vi "Make HTTP Request v4.vi"(0 "HTTP-Verb":string(combo)="GET", 3 "URL Prefix":string, 4 "URL Suffix":string, 5 "error in":errorcluster, 6 "request headers":T1[](array[typedef])=[{"name"="Content-Type", "value"="application/x-amz-json-1.1"}], 7 "request parameters":T1[](array[typedef]), 9 "request body":string, 10 "AWS Core":refnum<class "NI_AWS_Core.lvclass">) -> (12 "Call Result":string, 14 "response headers":string, 16 "response body":string, 19 "error out":errorcluster)   [LabVIEW 2015, in "NI_AWS_Core.lvclass"]
uses:
  NI_AWS_Core.lvclass
  Name Value Pair.ctl
  NI_AWS_Core.lvclass/NI_AWS_Core.ctl
  Read Credentials.vi
  Read Service.vi
  Read Region.vi
  Read Verify Server.vi
  <vilib>/httpClient/LabVIEWHTTPClient.lvlib
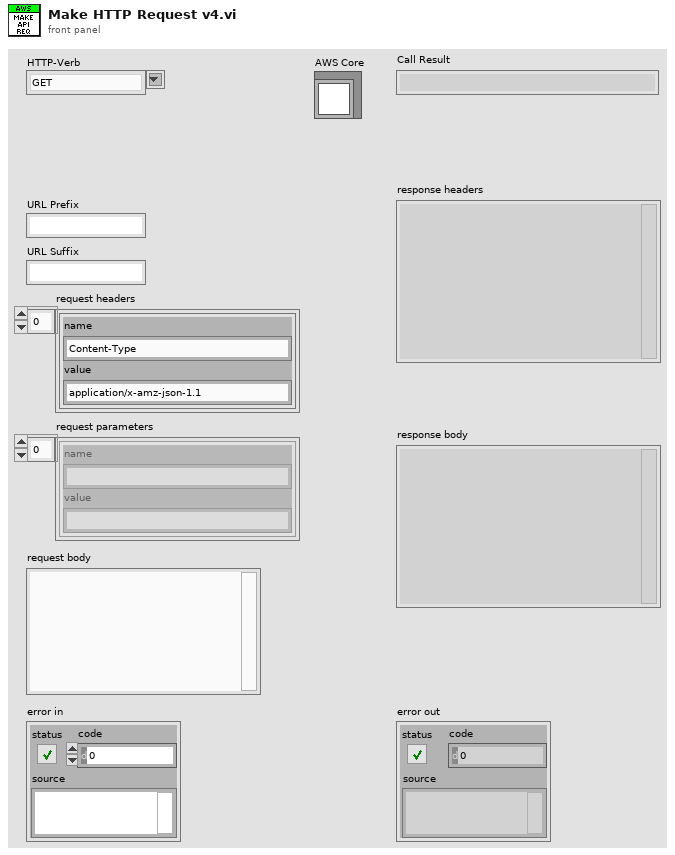
[diagram p1: front panel]
types:
  T1 = typedef "NI_AWS_Core.lvclass/Name Value Pair.ctl" = cluster{"name":string, "value":string}
  T2 = typedef "AWS Core.lvlib/AWS Credentials.ctl" = cluster{"Access Key":string, "Secret Key":string}
  T3 = typedef "NI_AWS Core.lvlib/Region.ctl" = enum16{"us-east-1", "us-east-2", "us-west-1", "us-west-2", "ap-northeast-1", "ap-northeast-2", "ap-southeast-1", "ap-southeast-2", "ca-central-1", "eu-central-1", "eu-west-1", "eu-west-2", "sa-east-1"}
  T4 = typedef "LabVIEWHTTPClient.lvlib/ClientHandle.ctl" = refnum<k1>
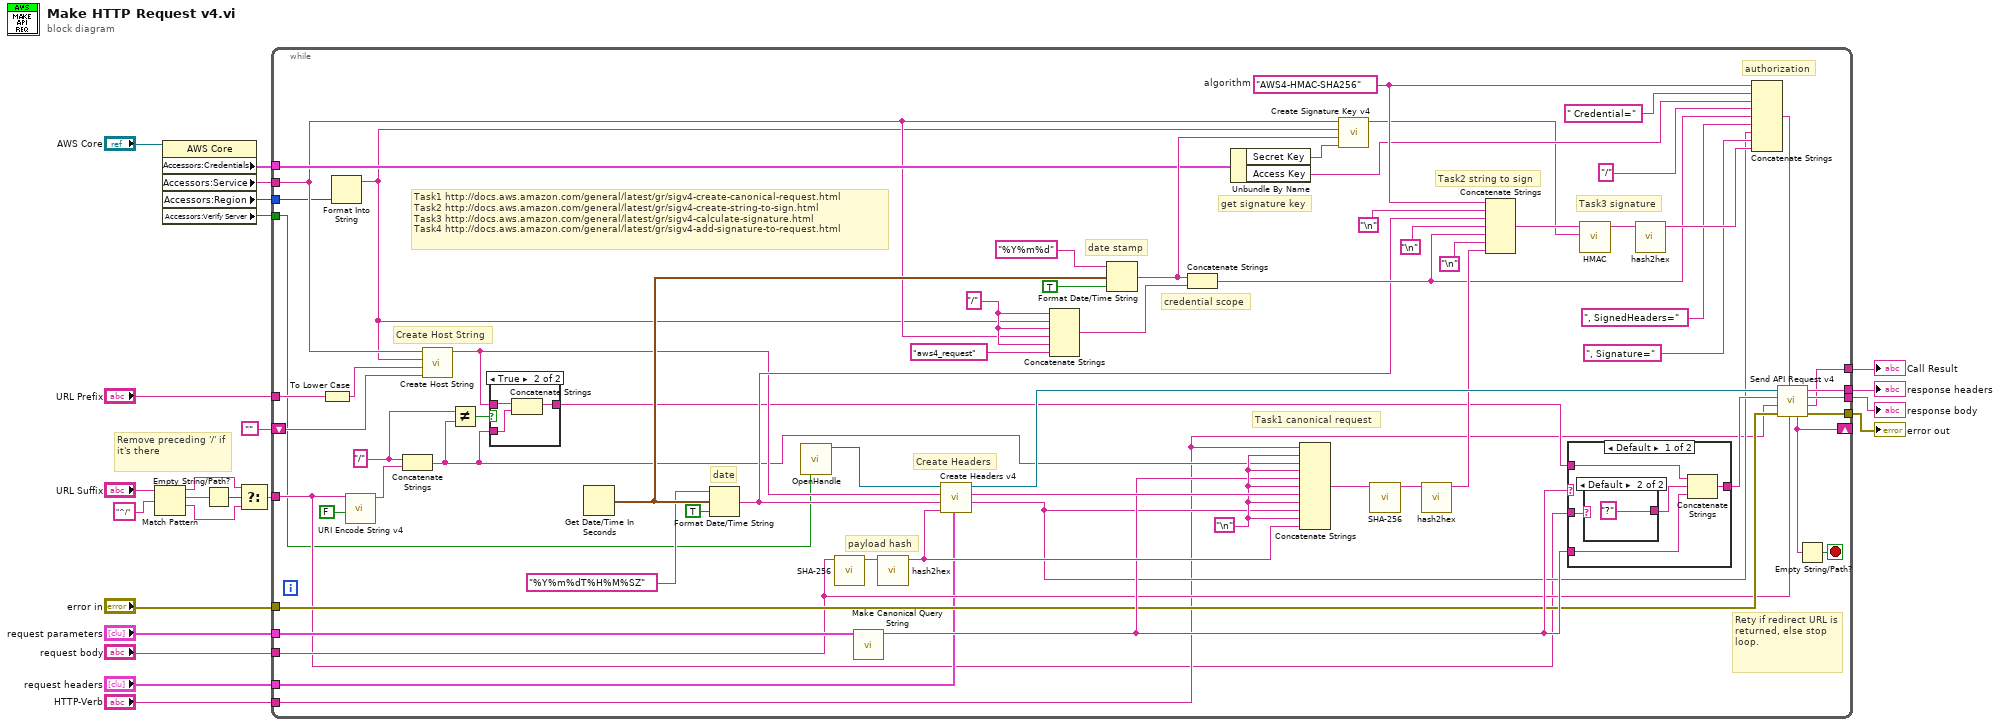
[diagram p0: block diagram]
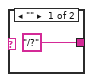
[diagram p3: hidden frame]
diagram:
  # "Remove preceding '/' if it's there"
  n1 = Match Pattern(string="URL Suffix", regular expression="^/") -> (before substring=w17:string, match substring=w15:string, after substring=w18:string)  [unwired: 1 in, 1 out]
  n2 = property class="AWS Core"(reference="AWS Core") -> ("Accessors:Credentials"=w5:T2, "Accessors:Service"=w3:string, "Accessors:Region"=w2:T3, "Accessors:Verify Server"=w1:bool)  [unwired: 1 in, 2 out]
  n3 = Empty String/Path?(string/path=w15) -> (empty?=w16:bool)
  n4 = Select(t=w17, s=w16, f=w18) -> (s? t:f=w13:string)
  n5 = while {
    tunnel: [w88] -> w23
    tunnel: [w41] -> w21
    tunnel: [w46] -> w20
    shift-right: [w45] -> _
    shift-left: "" ("Redirect endpoint") -> [w43]
    tunnel: [w42] -> w22
    tunnel: "error in" -> [w38]
    tunnel: w13 -> [w28]
    tunnel: "URL Prefix" -> [w34]
    tunnel: "request parameters" -> [w33]
    tunnel: "request body" -> [w32]
    tunnel: "request headers" -> [w31]
    tunnel: "HTTP-Verb" -> [w30]
    tunnel: w5 -> [w29]
    tunnel: w3 -> [w27]
    tunnel: w2 -> [w25]
    tunnel: w1 -> [w26]
    stop <- w44 stop-if-true
    w51 = "/" ("string")
    w62 = "/" ("string")
    w80 = "AWS4-HMAC-SHA256"  # algorithm
    w58 = "\n"
    # "Rety if redirect URL is returned, else stop loop."
    # "Create Host String"
    # "Task1 canonical request"
    # "Create Headers"
    # "get signature key"
    # "Task1 http://docs.aws.amazon.com/general/latest/gr/sigv4-create-canonical-request.html\nTask2 http://docs.aws.amazon.com/general/latest/gr/sigv4-create-string-to-sign.html\nTask3 http://docs.aws.amazon.com/general/latest/gr/sigv4-calculate-signature.html\nTask4 http://docs.aws.amazon.com/general/latest/gr/sigv4-add-signature-to-request.html"
    # "date stamp"
    # "date"
    # "payload hash"
    # "authorization"
    # "Task3 signature"
    # "Task2 string to sign"
    # "credential scope"
    n6 = To Lower Case(string=w34) -> (all lower case string=w39:string)
    n7 = Format Into String(w25) -> (resulting string=w24:string)  [unwired: 3 in, 1 out]
    n8 = call "URI Encode String v4.vi"("Encode /"=FALSE, "Un-encoded String"=w28) -> ("UriEncoded String"=w36:string)  [unwired: 9 in]
    n9 = Concatenate Strings(w51, w36) -> (w48:string)
    n10 = call "Create Host String.vi"("Redirect Endpoint"=w43, "URL Prefix"=w39, "Region"=w24, "AWS Service"=w27) -> ("Host String"=w49:string)  [unwired: 7 in]
    n11 = Not Equal?(x=w51, y=w48) -> (x != y?=w50:bool)
    n12 = case shown="True" w50 {
      tunnel: w49 -> [w89 w92]
      tunnel: w48 -> [_ w91]
      tunnel: [w89 w90] -> w47
      frame False {
      }
      frame True {
        n13 = Concatenate Strings(w92, w91) -> (w90:string)
      }
    }
    n14 = Get Date/Time In Seconds() -> (seconds since 1Jan1904=w55:timestamp)
    n15 = Format Date/Time String(time format string (%c)="%Y%m%dT%H%M%SZ", seconds (now)=w55, UTC format=TRUE) -> (date/time string=w56:string)
    n16 = call <vilib>:"OpenHandle.vi"("verify server(true)"=w26) -> ("client handle out"=w59:T4)  [unwired: 13 in, 1 out]
    n17 = call "SHA-256.vi"("Message"=w32) -> ("Hash Value"=w72:string)  [unwired: 10 in]
    n18 = call "Make Canonical Query String.vi"("request parameters"=w33) -> ("canonical parameters"=w52:string)  [unwired: 10 in]
    n19 = call "hash2hex.vi"("hash string"=w72) -> ("hex string"=w57:string)  [unwired: 10 in]
    n20 = call "Create Headers v4.vi"("request headers"=w31, "RequestBody Payload"=w57, "date/time string"=w56, "Host"=w49, "Client Handle In"=w59) -> ("Signed Headers"=w40:string, "canonical headers"=w76:string, "Client Handle Out"=w86:T4)  [unwired: 3 in]
    n21 = Concatenate Strings(w62, w24, w62, w27, w62, "aws4_request" ("string")) -> (w63:string)
    n22 = Format Date/Time String(time format string (%c)="%Y%m%d", seconds (now)=w55, UTC format=TRUE) -> (date/time string=w69:string)
    n23 = Concatenate Strings(w69, w63) -> (w64:string)
    n24 = Unbundle By Name(w29) -> ("Secret Key"=w60:string, "Access Key"=w66:string)
    n25 = Concatenate Strings(w30, w58, w48, w58, w52, w58, w76, w58, w40, w58, w57) -> (w71:string)
    n26 = call "Create Signature Key v4.vi"("AWS Service"=w27, "Region"=w24, "date/time string"=w69, "Secret Key"=w60) -> ("Keyed-Hash"=w37:string)  [unwired: 6 in]
    n27 = call "SHA-256.vi"("Message"=w71) -> ("Hash Value"=w70:string)  [unwired: 10 in]
    n28 = call "hash2hex.vi"("hash string"=w70) -> ("hex string"=w79:string)  [unwired: 10 in]
    n29 = Concatenate Strings(w80, "\n", w56, "\n", w64, "\n", w79) -> (w68:string)
    n30 = case shown="Default" w52 {
      tunnel: [w97 w100] -> w53
      tunnel: w47 -> [w95 w100]
      tunnel: w52 -> [w96 _]
      tunnel: w28 -> [w93 _]
      frame Default {
        n31 = case shown="Default" w93 {
          tunnel: ["/?" ("string") "?" ("string")] -> w94
          frame "" {
          }
          frame Default {
          }
        }
        n32 = Concatenate Strings(w95, w94, w96) -> (w97:string)
      }
      frame "" {
      }
    }
    n33 = call "HMAC.vi"("Key"=w37, "Message"=w68) -> ("Keyed Hash"=w67:string)  [unwired: 9 in]
    n34 = call "hash2hex.vi"("hash string"=w67) -> ("hex string"=w85:string)  [unwired: 10 in]
    n35 = Concatenate Strings(w80, " Credential=", w66, "/", w64, ", SignedHeaders=", w40, ", Signature=", w85) -> (w87:string)
    n36 = call "Send API Request v4.vi"("request body"=w32, "Authorization"=w87, "error in (no error)"=w38, "HTTP-Verb"=w30, "Host String"=w53, "Client Handle"=w86) -> ("error out"=w41:errorcluster, "Call Result"=w42:string, "response body"=w46:string, "response headers"=w88:string, "Redirect endpoint"=w45:string)  [unwired: 1 in]
    n37 = Empty String/Path?(string/path=w45) -> (empty?=w44:bool)
  }
  "response headers" <- w23
  "response body" <- w20
  "error out" <- w21
  "Call Result" <- w22
